vi "get pixel clock range.vi"(8 "error in (no error)":errorcluster, 11 "Thorcam in":refnum<class "Thorcam.lvclass">) -> (0 "error out":errorcluster, 3 "Thorcam out":refnum<class "Thorcam.lvclass">)   [LabVIEW 2012, in "Thorcam.lvclass"]
uses:
  Thorcam.lvclass
  Thorcam.lvclass/Thorcam.ctl
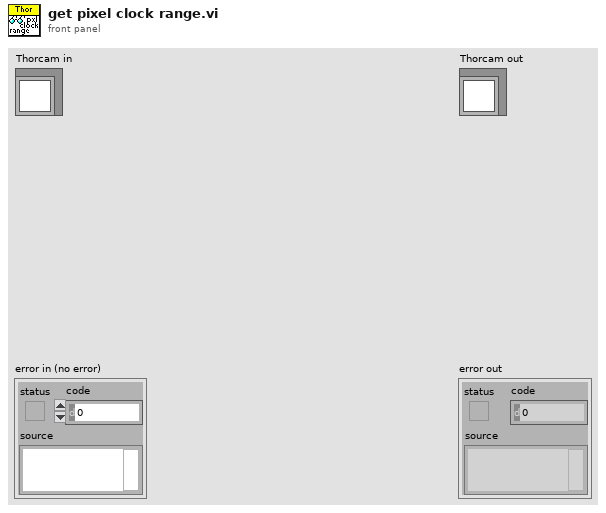
[diagram p1: front panel]
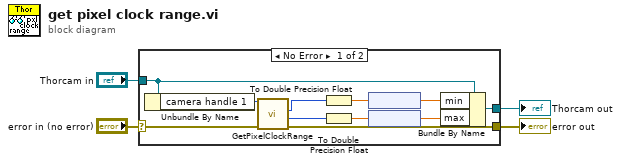
[diagram p0: block diagram]
diagram:
  n1 = case shown="No Error" "error in (no error)" {
    selector: "error in (no error)" -> [w14 w17]
    tunnel: [w13 w17] -> w3
    tunnel: [w9 w16] -> w1
    tunnel: "Thorcam in" -> [w10 w16]
    frame No Error {
      n2 = Unbundle By Name(w10) -> ("camera handle 1"=w15:u32)
      n3 = call <instrlib>:"GetPixelClockRange.vi"("error in"=w14, "Camera Handle In"=w15) -> ("error out"=w13:errorcluster, "Max"=w11:i32, "Min"=w12:i32)  [unwired: 6 in, 1 out]
      n4 = To Double Precision Float(number=w12) -> (double precision float=w6:dbl)
      n5 = To Double Precision Float(number=w11) -> (double precision float=w5:dbl)
      n6 = node(w6) -> (w8:dbl[unit])
      n7 = node(w5) -> (w7:dbl[unit])
      n8 = Bundle By Name(cluster=w10, "min"=w8, "max"=w7) -> (w9:refnum<class "Thorcam.lvclass">)
    }
    frame Error {
    }
  }
  "error out" <- w3
  "Thorcam out" <- w1
